vi "back_to_EOL_symbols.vi"(8 "error in (no error)":errorcluster, 11 "value":string) -> (0 "error out":errorcluster, 3 "result string":string)   [LabVIEW 2015, in "ini_work_Library.lvlib"]
doc: "Replaxes /n symbol to EOL constant\nCreated by Artem Shevelev\nshevelev.pro\nartem@shevelev.pro\nLabVIEW Portal: https://labviewportal.org/memberlist.php?mode=viewprofile&u=2340"
uses:
  ini_work_Library.lvlib
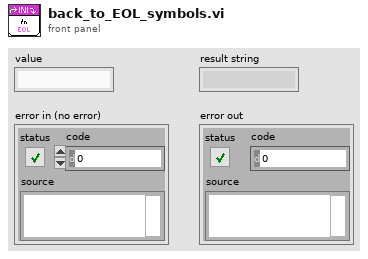
[diagram p1: front panel]
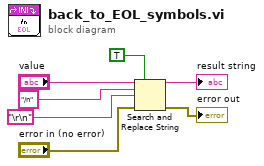
[diagram p0: block diagram]
diagram:
  n1 = Search and Replace String(replace all?=TRUE ("replace all? (F)"), input string="value", search string="/n" ("replace string (\"\")"), replace string="\r\n", error in="error in (no error)") -> (result string=→"result string":string, error out=→"error out":errorcluster)  [unwired: 3 in, 2 out]
